vi "Check Number In Middle E-Series.vi"(8 "1D sel":T1, 9 "2D sel":T1, 10 "3D sel":T1, 11 "E Serie":u16[](array[numeric])) -> (3 "In Serie?":bool)   [LabVIEW 2018]
uses:
  digit--enum.ctl
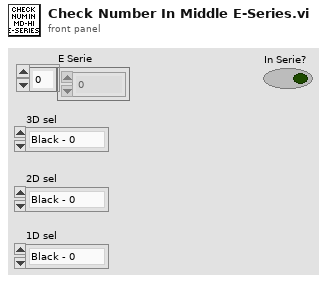
[diagram p1: front panel]
types:
  T1 = typedef "digit--enum.ctl" = enum16{"Black - 0", "Brown - 1", "Red - 2", "Orange - 3", "Yellow - 4", "Green - 5", "Blue - 6", "Violet - 7", "Grey - 8", "White - 9"}
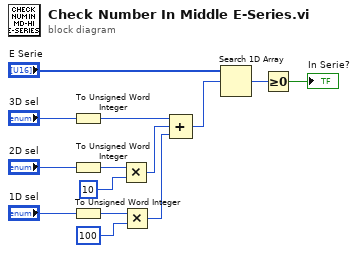
[diagram p0: block diagram]
diagram:
  n1 = To Unsigned Word Integer(number="3D sel") -> (unsigned 16bit integer=w3:u16)
  n2 = To Unsigned Word Integer(number="2D sel") -> (unsigned 16bit integer=w6:u16)
  n3 = To Unsigned Word Integer(number="1D sel") -> (unsigned 16bit integer=w9:u16)
  n4 = Multiply(x=w6, y=u16 10) -> (x*y=w2:u16)
  n5 = Multiply(x=w9, y=u16 100) -> (x*y=w1:u16)
  n6 = Compound Arithmetic op=ADD(w3, w2, w1) -> (w12:u16)
  n7 = Search 1D Array(1D array="E Serie", element=w12) -> (index of element=w13:i32)  [unwired: 1 in]
  n8 = Greater Or Equal To 0?(x=w13) -> (x >= 0?=→"In Serie?":bool)
